vi "超标浓度设置.vi"(11 "输入":T1) -> (3 "输出":T2)   [LabVIEW 2016, in "德润DR803M超标留样.lvlib"]
uses:
  <vilib>/Utility/miscctls.llb/LVPointTypeDef.ctl
panel:
  in  "取消":bool
  in  "确定":bool
  in  "CODCr超标浓度":dbl
  in  "CODMn超标浓度":dbl
  in  "总氮超标浓度":dbl
  in  "总磷超标浓度":dbl
  in  "氨氮超标浓度":dbl
  # "超标浓度报警配置"
  # "mg/L"
  # "mg/L"
  # "mg/L"
  # "mg/L"
  # "mg/L"
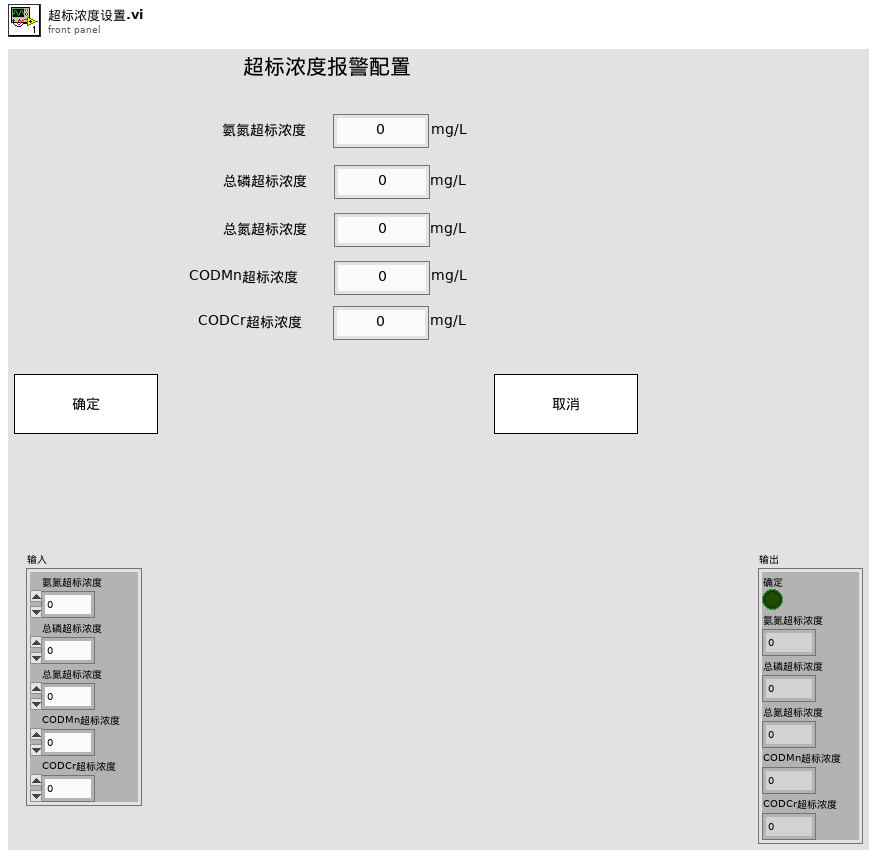
[diagram p1: front panel]
types:
  T1 = cluster{"氨氮超标浓度":dbl, "总磷超标浓度":dbl, "总氮超标浓度":dbl, "CODMn超标浓度":dbl, "CODCr超标浓度":dbl}
  T2 = cluster{"确定":bool, "氨氮超标浓度":dbl, "总磷超标浓度":dbl, "总氮超标浓度":dbl, "CODMn超标浓度":dbl, "CODCr超标浓度":dbl}
  T3 = typedef "LVPointTypeDef.ctl" = cluster{"Horizontal":i16, "Vertical":i16}
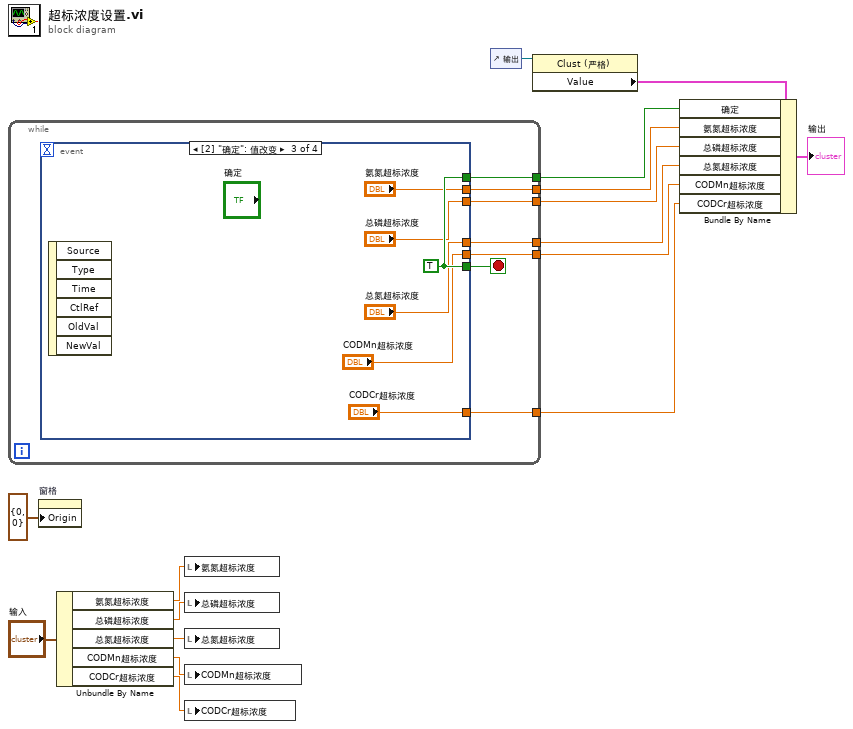
[diagram p0: block diagram]
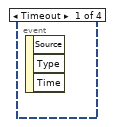
[diagram p2: hidden frame]
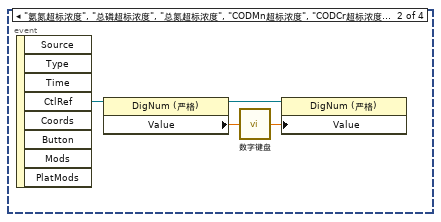
[diagram p3: hidden frame]
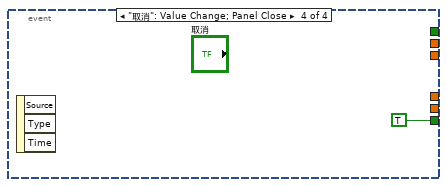
[diagram p4: hidden frame]
diagram:
  n1 = while {
    tunnel: [w22] -> w13
    tunnel: [w21] -> w12
    tunnel: [w20] -> w11
    tunnel: [w19] -> w10
    tunnel: [w18] -> w9
    tunnel: [w17] -> w8
    stop <- w23 stop-if-true
    n2 = event shown="[2] \"确定\": 值改变" {
      selector: _ -> [_ _ _ _]
      dyn-events: _ -> [_ _ _ _]
      timeout: _ -> [_ _ _ _]
      tunnel: [_ _ w33 TRUE] -> w23
      tunnel: [_ _ w33 _] -> w22
      tunnel: [_ _ "氨氮超标浓度" _] -> w21
      tunnel: [_ _ "总磷超标浓度" _] -> w20
      tunnel: [_ _ "总氮超标浓度" _] -> w19
      tunnel: [_ _ "CODMn超标浓度" _] -> w18
      tunnel: [_ _ "CODCr超标浓度" _] -> w17
      event Timeout {
        n3 = event-data() -> ()  [unwired: 1 in, 3 out]
      }
      event "氨氮超标浓度", "总磷超标浓度", "总氮超标浓度", "CODMn超标浓度", "CODCr超标浓度": Mouse Down {
        n4 = event-data() -> ("CtlRef"=w27:refnum<vi>)  [unwired: 1 in, 7 out]
        n5 = property class="DigNum (严格)"(reference=w27) -> (reference out=w25:refnum<vi>, "Value"=w26:dbl)  [unwired: 1 in, 1 out]
        n6 = call "数字键盘.vi"("OldNumber"=w26) -> ("NewNumber"=w24:sgl)
        n7 = property class="DigNum (严格)"(reference=w25, "Value"=w24) -> ()  [unwired: 1 in, 2 out]
      }
      event "确定": Value Change {
        w33 = TRUE
        n8 = event-data() -> ()  [unwired: 1 in, 6 out]
      }
      event "取消": Value Change; Panel Close {
        n9 = event-data() -> ()  [unwired: 1 in, 3 out]
      }
    }
  }
  n10 = property on="窗格" class="Pane"("Origin"=T3 {"Horizontal"=0, "Vertical"=0} ("原点")) -> ()  [unwired: 2 in, 2 out]
  n11 = Unbundle By Name("输入") -> ("氨氮超标浓度"=w6:dbl, "总磷超标浓度"=w5:dbl, "总氮超标浓度"=w4:dbl, "CODMn超标浓度"=w3:dbl, "CODCr超标浓度"=w2:dbl)
  n12 = local write "氨氮超标浓度"(w6) -> ()
  n13 = local write "总磷超标浓度"(w5) -> ()
  n14 = local write "总氮超标浓度"(w4) -> ()
  n15 = local write "CODMn超标浓度"(w3) -> ()
  n16 = local write "CODCr超标浓度"(w2) -> ()
  n17 = control-ref of="输出"() -> (w16:refnum<vi>)
  n18 = property class="Clust (严格)"(reference=w16) -> ("Value"=w15:T2)  [unwired: 1 in, 2 out]
  n19 = Bundle By Name(cluster=w15, "确定"=w13, "氨氮超标浓度"=w12, "总磷超标浓度"=w11, "总氮超标浓度"=w10, "CODMn超标浓度"=w9, "CODCr超标浓度"=w8) -> (→"输出":T2)
